vi "Initialize.vi"(8 "error in":errorcluster, 11 "Modbus slave in":refnum<class "Modbus Slave.lvclass">) -> (0 "error out":errorcluster, 3 "Modbus slave out":refnum<class "Modbus Slave.lvclass">)   [LabVIEW 2012, in "Modbus Slave.lvclass"]
doc: "Initializes a Modbus slave instance. If using the <B>Create Modbus Instance</B> VI, this is not necessary. This function will initiate any required bus communication and launch a daemon to handle incoming requests from the master."
uses:
  Modbus Slave.lvclass
  Modbus Slave.lvclass/Modbus Slave.ctl
  Modbus API.lvclass/Modbus API.ctl
  Data Model/Device Data Model.lvclass
  Network Protocol/Network Slave/Network Slave.lvclass
  Modbus API.lvclass
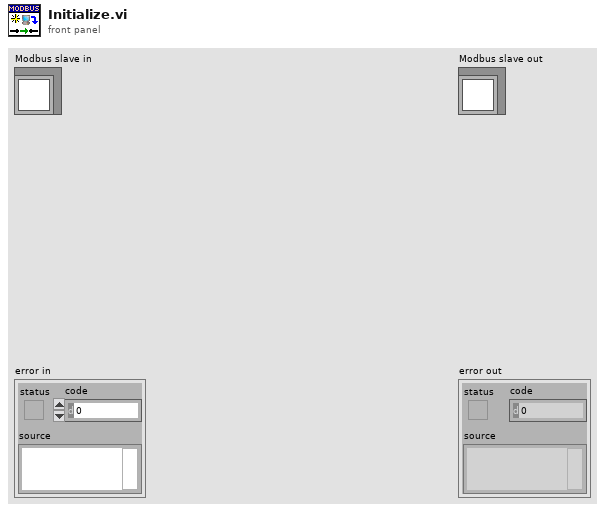
[diagram p1: front panel]
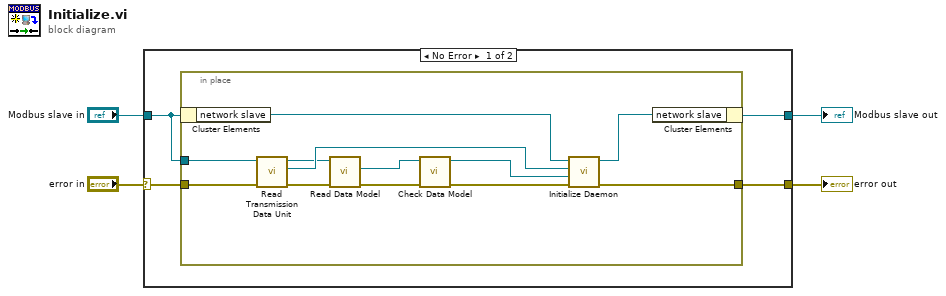
[diagram p0: block diagram]
diagram:
  n1 = case shown="No Error" "error in" {
    selector: "error in" -> [w6 w22]
    tunnel: [w5 w21] -> w4
    tunnel: "Modbus slave in" -> [w7 w21]
    tunnel: [w8 w22] -> w2
    frame No Error {
      n2 = in-place {
        in-place-border: [w20] -> w8
        in-place-border: w7 -> [w11]
        in-place-border: w6 -> [w12]
        n3 = in-place-cluster #1(w7) -> ("network slave"=w9:refnum<class "Network Slave.lvclass">)
        n4 = call "Read Transmission Data Unit.vi"("error in"=w12, "Modbus instance in"=w11) -> ("error out"=w13:errorcluster, "transmission data unit"=w16:refnum<class "Transmission Data Unit.lvclass">, "Modbus instance out"=w14:refnum<class "Modbus Slave.lvclass">)  [unwired: 7 in]
        n5 = call "Read Data Model.vi"("error in"=w13, "Modbus slave in"=w14) -> ("error out"=w10:errorcluster, "Device Data Model"=w15:refnum<class "Device Data Model.lvclass">)  [unwired: 7 in, 1 out]
        n6 = call-dynamic "Check Data Model.vi"("error in"=w10, "device data model in"=w15) -> ("error out"=w19:errorcluster, "device data model out"=w17:refnum<class "Device Data Model.lvclass">)  [unwired: 8 in]
        n7 = call-dynamic "Initialize Daemon.vi"("error in"=w19, "Data Model"=w17, "transmission data unit"=w16, "network slave in"=w9) -> ("error out"=w20:errorcluster, "network slave out"=w18:refnum<class "Network Slave.lvclass">)  [unwired: 6 in]
        n8 = in-place-cluster #1("network slave"=w18) -> (w5:refnum<class "Modbus Slave.lvclass">)
      }
    }
    frame Error {
    }
  }
  "error out" <- w2
  "Modbus slave out" <- w4
